vi "Insert Down SubPanel.vi"(8 "error in (no error)":errorcluster, 9 "ActorQName":string, 10 "ActorVI Ref":refnum<vi>, 11 "UI_Up_Down in":refnum<class "Model_AMC.lvclass">) -> (0 "error out":errorcluster, 3 "UI_Up_Down out":refnum<class "Model_AMC.lvclass">)   [LabVIEW 2021]
uses:
  <vilib>/ActorFramework/Actor/Actor.lvclass
  <userlib>/John_Lib/AbstractActorTemplate/UIActorTop Messages/UI Initialize Msg/UI Initialize Msg.lvclass
  Model_AMC.lvclass
  C:/Program Files (x86)/National Instruments/LabVIEW 2021/user.lib/John_Lib/AbstractActorTemplate/AbstractActorTemplate/UIActorTop.lvclass
  C:/Program Files (x86)/National Instruments/LabVIEW 2021/vi.lib/ActorFramework/Actor/Actor.lvclass
  C:/Program Files (x86)/National Instruments/LabVIEW 2021/project/Create Actor from Template/_Model_AMC/Model_AMC.lvclass
  C:/Program Files (x86)/National Instruments/LabVIEW 2021/user.lib/John_Lib/Interfaces/InsertUpDownSubPanel/InsertUpDownSubPanel.lvclass
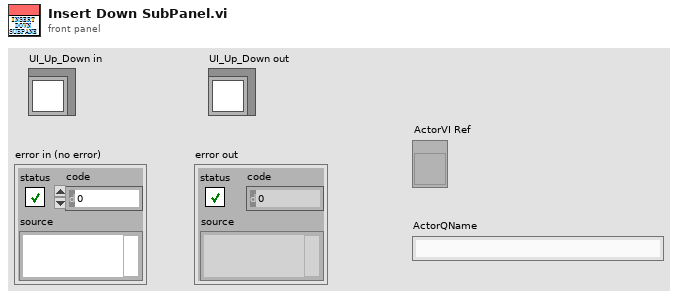
[diagram p1: front panel]
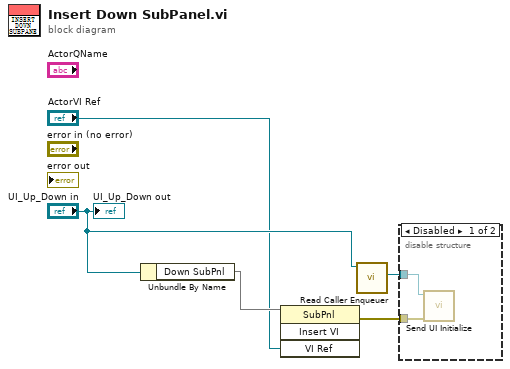
[diagram p0: block diagram]
diagram:
  n1 = Unbundle By Name("UI_Up_Down in") -> ("Down SubPnl"=w3)
  n2 = invoke class="SubPnl" method="Insert VI"(reference=w3, "VI Ref"="ActorVI Ref") -> (error out=w5:errorcluster)  [unwired: 2 in, 3 out]
  n3 = call <vilib>:"Read Caller Enqueuer.vi"("Actor"="UI_Up_Down in") -> ("Caller Enqueuer"=w4:refnum<class "Message Enqueuer.lvclass">)  [unwired: 10 in]
  n4 = disable-structure shown="Disabled" {
    disable-tunnel: w5 -> [w7 _]
    disable-tunnel: w4 -> [w6 _]
    frame Disabled {
      n5 = call <userlib>:"Send UI Initialize.vi"("error in (no error)"=w7, "Message Enqueuer"=w6) -> ()  [unwired: 8 in, 2 out]
    }
    frame Enabled {
    }
  }
  "UI_Up_Down out" <- "UI_Up_Down in"
